vi "Channel Specification.vi"(8 "error in":errorcluster, 11 "Node Ptr":T1 format="%.0x") -> (0 "error out":errorcluster)   [LabVIEW 2024, in "AIM ARINC 429 System Explorer.lvlib" / "Implementation.lvlib"]
uses:
  Implementation.lvlib
  <vilib>/NI VeriStand/Custom Device API/Custom Device Item Ref.ctl
  Scripting/AIM/Constants.vi
  <vilib>/NI VeriStand/Custom Device API/Custom Device API.lvlib
  Scripting/AIM/AIM ARINC 429 Scripting.lvlib
panel:
  out "Channel Settings":string[][](table)=[["Type", "Input"], ["Units", ""], ["Default Value", "0.000000"], ["Faultable", "No"], ["Scalable", "No"]]
  in  "Default Value":dbl
  in  "SHDocVw.IWebBrowser":refnum<k7>(container)
  in  "General Header":cluster{"Section Name":string}={"Section Name"="ARINC 429 - Channel Specification"}
  in  "Description":string
  out "Name":string
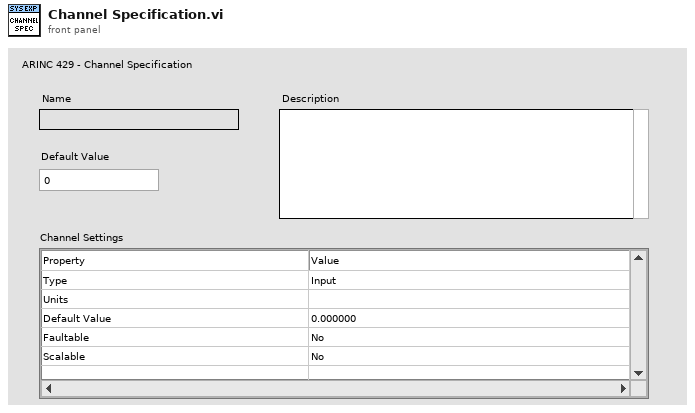
[diagram p1: front panel]
types:
  T1 = typedef "Custom Device API.lvlib/Custom Device Item Ref.ctl" = u64
  T2 = typedef "Custom Device API.lvlib/Custom Device Channel.ctl" = cluster{"Type":T3, "Units":string, "Default Value":dbl, "Faultable":bool, "Scalable":bool}
  T3 = typedef "Custom Device API.lvlib/Custom Device Channel Type.ctl" = enum16{"Input", "Output"}
  T4 = typedef "Custom Device API.lvlib/Custom Device Item Info.ctl" = cluster{"Name":string, "Is Channel":bool, "GUID":string, "Is Waveform":bool}
  T5 = typedef "Custom Device API.lvlib/Custom Device Commands.ctl" = enum16{"Default", "Item renamed", "Shutdown", "Dynamic button pressed"}
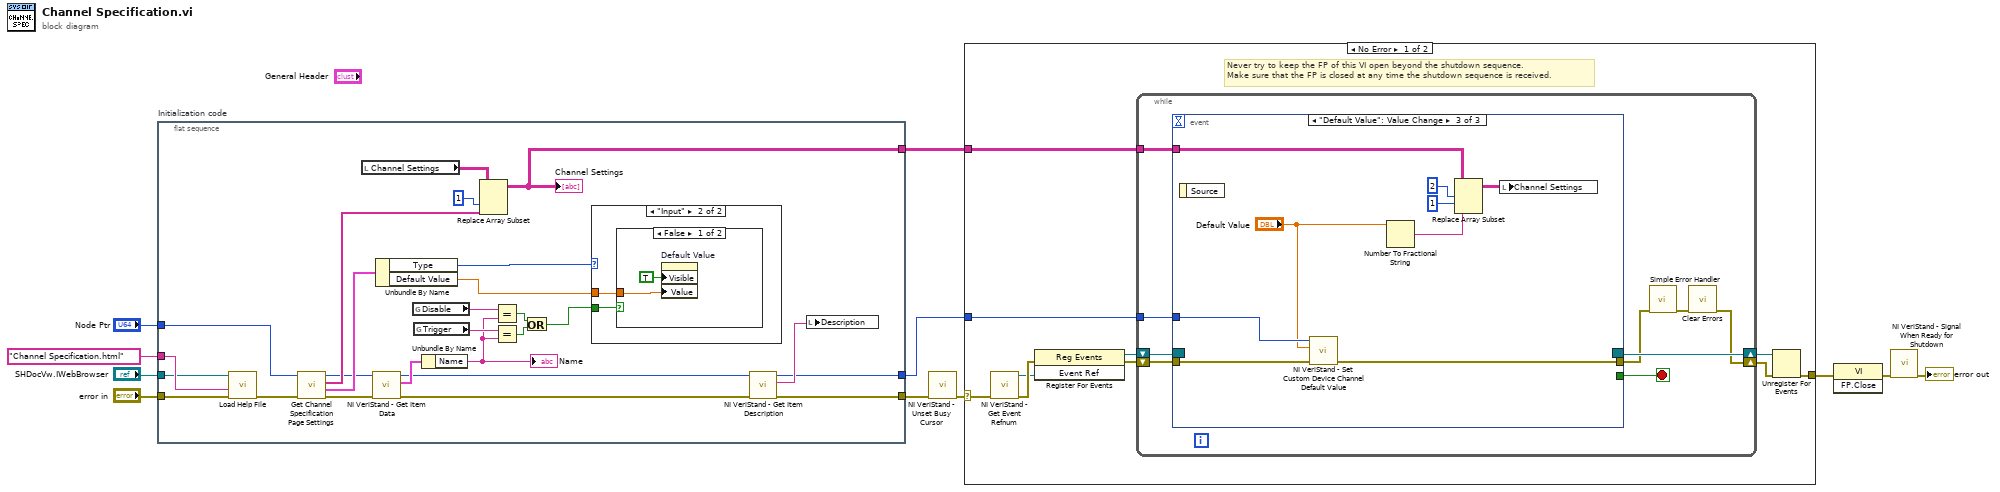
[diagram p0: block diagram]
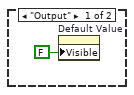
[diagram p2: hidden frame]
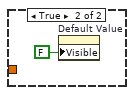
[diagram p3: hidden frame]
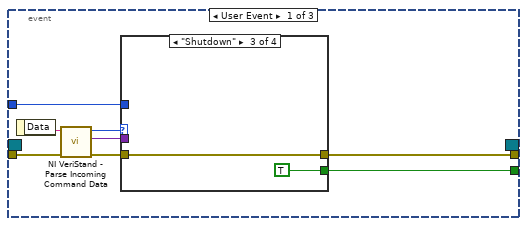
[diagram p4: hidden frame]
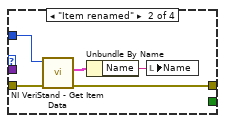
[diagram p6: hidden frame]
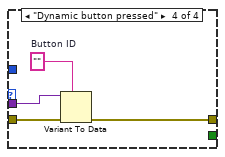
[diagram p7: hidden frame]
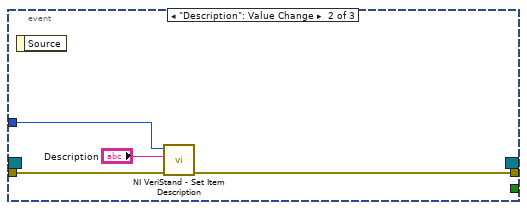
[diagram p8: hidden frame]
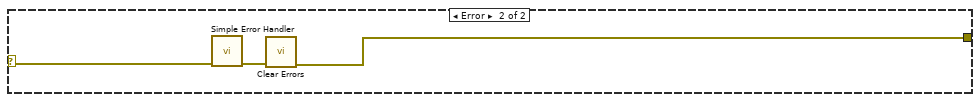
[diagram p9: hidden frame]
diagram:
  n1 = flat-sequence "Initialization code" {
    tunnel: "error in" -> [w35]
    tunnel: "Node Ptr" -> [w29]
    tunnel: [w19] -> w7
    tunnel: [w20] -> w4
    tunnel: "SHDocVw.IWebBrowser" -> [w33]
    tunnel: "Channel Specification.html" ("CD_CHM_Section") -> [w34]
    tunnel: [w24] -> w1
    frame #0 {
      n2 = call "Load Help File.vi"("error in (no error)"=w35, "HTML File to Load"=w34, "Browser"=w33) -> ("error out"=w28:errorcluster)  [unwired: 8 in]
      n3 = call "Get Channel Specification Page Settings.vi"("error in"=w28, "parameter ref"=w29) -> ("error out"=w22:errorcluster, "Channel"=w26:T2, "Channel Settings"=w25:string[], "parameter ref out"=w23:T1)  [unwired: 6 in]
      n4 = local read "Channel Settings"() -> (w32:string[][])
      n5 = call <vilib>:"NI VeriStand - Get Item Data.vi"("error in (no error)"=w22, "Item Ref in"=w23) -> ("error out"=w18:errorcluster, "Item Info"=w37:T4, "Item Ref out"=w21:T1)  [unwired: 7 out]
      n6 = Unbundle By Name(w26) -> ("Type"=w30:T3, "Default Value"=w27:dbl)
      n7 = global read "Constants.vi" "Disable"() -> (w17:string)
      n8 = global read "Constants.vi" "Trigger"() -> (w16:string)
      n9 = Unbundle By Name(w37) -> ("Name"=w15:string)
      "Name" <- w15
      n10 = Replace Array Subset(array=w32, new element=w25, index (col)=1 ("disabled index (col)")) -> (w24:string[][])  [unwired: 1 in]
      "Channel Settings" <- w24
      n11 = Equal?(x=w17, y=w15) -> (x = y?=w14:bool)
      n12 = Equal?(x=w16, y=w15) -> (x = y?=w13:bool)
      n13 = Or(x=w14, y=w13) -> (x .or. y?=w12:bool)
      n14 = case shown="\"Input\"" w30 {
        tunnel: w27 -> [_ w40]
        tunnel: w12 -> [_ w39]
        frame "Output" {
          n15 = property on="Default Value" class="DigNum (strict)"("Visible"=FALSE) -> ()  [unwired: 2 in, 2 out]
        }
        frame "Input" {
          n16 = case shown="False" w39 {
            tunnel: w40 -> [w42 _]
            frame False {
              n17 = property on="Default Value" class="DigNum (strict)"("Visible"=TRUE, "Value"=w42) -> ()  [unwired: 2 in, 2 out]
            }
            frame True {
              n18 = property on="Default Value" class="DigNum (strict)"("Visible"=FALSE) -> ()  [unwired: 2 in, 2 out]
            }
          }
        }
      }
      n19 = call <vilib>:"NI VeriStand - Get Item Description.vi"("error in (no error)"=w18, "Item Ref in"=w21) -> ("error out"=w19:errorcluster, "Description"=w36:string, "Item Ref out"=w20:T1)  [unwired: 7 out]
      n20 = local write "Description"(w36) -> ()
    }
  }
  n21 = call <vilib>:"NI VeriStand - Unset Busy Cursor.vi"("error in (no error)"=w7) -> ("error out"=w6:errorcluster)  [unwired: 10 out]
  n22 = case shown="No Error" w6 {
    selector: w6 -> [w45 w98]
    tunnel: [w50 w96] -> w11
    tunnel: w4 -> [w46 _]
    tunnel: w1 -> [w44 _]
    frame No Error {
      # "Never try to keep the FP of this VI open beyond the shutdown sequence.\nMake sure that the FP is closed at any time the shutdown sequence is received."
      n23 = call <vilib>:"NI VeriStand - Get Event Refnum.vi"("error in (no error)"=w45) -> ("error out"=w53:errorcluster, "Event Ref"=w49:refnum<user-event>)  [unwired: 9 out]
      n24 = register-events(error in=w53, w49) -> (reference out=w47:refnum<event-registration>, error out=w48:errorcluster)  [unwired: 1 in]
      n25 = while {
        tunnel: w46 -> [w58]
        shift-right: [w55] -> w51
        shift-left: w48 -> [w61]
        shift-right: [w62] -> w52
        shift-left: w47 -> [w60]
        tunnel: w44 -> [w54]
        stop <- w59 stop-if-true
        n26 = event shown="[2] \"Default Value\": Value Change" {
          selector: w60 -> [_ _ _]
          dyn-events: [_ _ _] -> w62
          timeout: _ -> [_ _ _]
          tunnel: w61 -> [w70 w85 w94]
          tunnel: [w66 _ _] -> w59
          tunnel: [w65 w84 w93] -> w57
          tunnel: w58 -> [w64 w86 w95]
          tunnel: w54 -> [_ _ w92]
          event User Event {
            n27 = event-data() -> ("Data"=w69:string)  [unwired: 1 out]
            n28 = call <vilib>:"NI VeriStand - Parse Incoming Command Data.vi"("error in (no error)"=w70, "Incoming data"=w69) -> ("error out"=w68:errorcluster, "Outgoing data"=w63:variant, "Action"=w67:T5)  [unwired: 7 out]
            n29 = case shown="\"Shutdown\"" w67 {
              tunnel: w68 -> [w71 w76 w77 w82]
              tunnel: [_ _ TRUE _] -> w66
              tunnel: [w71 w73 w77 w79] -> w65
              tunnel: w64 -> [_ w75 _ _]
              tunnel: w63 -> [_ _ _ w81]
              frame "Default", Default {
              }
              frame "Item renamed" {
                n30 = call <vilib>:"NI VeriStand - Get Item Data.vi"("error in (no error)"=w76, "Item Ref in"=w75) -> ("error out"=w73:errorcluster, "Item Info"=w74:T4)  [unwired: 8 out]
                n31 = Unbundle By Name(w74) -> ("Name"=w72:string)
                n32 = local write "Name"(w72) -> ()
              }
              frame "Shutdown" {
              }
              frame "Dynamic button pressed" {
                w80 = ""  # Button ID
                n33 = Variant To Data(error in=w82, type=w80, Variant=w81) -> (error out=w79:errorcluster)  [unwired: 1 out]
              }
            }
          }
          event "Description": Value Change {
            n34 = event-data() -> ()  [unwired: 2 out]
            n35 = call <vilib>:"NI VeriStand - Set Item Description.vi"("error in (no error)"=w85, "Description"="Description", "Item Ref in"=w86) -> ("error out"=w84:errorcluster)  [unwired: 8 out]
          }
          event "Default Value": Value Change {
            n36 = event-data() -> ()  [unwired: 2 out]
            n37 = call <vilib>:"NI VeriStand - Set Custom Device Channel Default Value.vi"("error in (no error)"=w94, "Default Value"="Default Value", "Channel Ref in"=w95) -> ("error out"=w93:errorcluster)  [unwired: 7 in, 1 out]
            n38 = Number To Fractional String(number="Default Value") -> (F-format string=w88:string)  [unwired: 3 in]
            n39 = Replace Array Subset(array=w92, new element=w88, index (row)=2, index (col)=1 ("disabled index (col)")) -> (w91:string[][])
            n40 = local write "Channel Settings"(w91) -> ()
          }
        }
        n41 = call <vilib>:"Simple Error Handler.vi"("error in (no error)"=w57) -> ("error out"=w56:errorcluster)  [unwired: 1 in, 7 out]
        n42 = call <vilib>:"Clear Errors.vi"("error in (no error)"=w56) -> ("error out"=w55:errorcluster)  [unwired: 1 in, 5 out]
      }
      n43 = Unregister For Events(event registration refnum=w52, error in=w51) -> (error out=w50:errorcluster)
    }
    frame Error {
      n44 = call <vilib>:"Simple Error Handler.vi"("error in (no error)"=w98) -> ("error out"=w97:errorcluster)  [unwired: 1 in, 7 out]
      n45 = call <vilib>:"Clear Errors.vi"("error in (no error)"=w97) -> ("error out"=w96:errorcluster)  [unwired: 1 in, 5 out]
    }
  }
  n46 = invoke class="VI" method="FP.Close"(error in=w11) -> (error out=w10:errorcluster)  [unwired: 2 in, 2 out]
  n47 = call <vilib>:"NI VeriStand - Signal When Ready for Shutdown.vi"("error in (no error)"=w10) -> ("error out"=→"error out":errorcluster)  [unwired: 10 out]
